vi "IMAQdx Errorcodes.vi"() -> ()   [LabVIEW 2014]
uses:
  <vilib>/Utility/error.llb/DialogType.ctl
panel:
  out "Array":errorcluster[](array[cluster])
  # "IMAQdxErrorSystemMemoryFull = 0xBFF69000,   // Not enough memory\n    IMAQdxErrorInternal,                        // Internal error\n    IMAQdxErrorInvalidParameter,                // Invalid parameter\n    IMAQdxErrorInvalidPointer,                  // Invalid pointer\n    IMAQdxErrorInvalidInterface,                // Invalid camera session\n    IMAQdxErrorInvalidRegistryKey,              // Invalid registry key\n    IMAQdxErrorInvalidAddress,                  // Invalid address\n    IMAQdxErrorInvalidDeviceType,               // Invalid device type\n    IMAQdxErrorNotImplemented,                  // Not implemented\n    IMAQdxErrorCameraNotFound,                  // Camera not found\n    IMAQdxErrorCameraInUse,                     // Camera is already in use.\n    IMAQdxErrorCameraNotInitialized,            // Camera is not initialized.\n    IMAQdxErrorCameraRemoved,                   // Camera has been removed.\n    IMAQdxErrorCameraRunning,                   // Acquisition in progress.\n    IMAQdxErrorCameraNotRunning,                // No acquisition in progress.\n    IMAQdxErrorAttributeNotSupported,           // Attribute not supported by the camera.\n    IMAQdxErrorAttributeNotSettable,            // Unable to set attribute.\n    IMAQdxErrorAttributeNotReadable,            // Unable to get attribute.\n    IMAQdxErrorAttributeOutOfRange,             // Attribute value is out of range.\n    IMAQdxErrorBufferNotAvailable,              // Requested buffer is unavailable.\n    IMAQdxErrorBufferListEmpty,                 // Buffer list is empty. Add one or more buffers.\n    IMAQdxErrorBufferListLocked,                // Buffer list is already locked. Reconfigure acquisition and try again.\n    IMAQdxErrorBufferListNotLocked,             // No buffer list. Reconfigure acquisition and try again.\n    IMAQdxErrorResourcesAllocated,              // Transfer engine resources already allocated. Reconfigure acquisition and try again.\n    IMAQdxErrorResourcesUnavailable,            // Insufficient transfer engine resources.\n    IMAQdxErrorAsyncWrite,                      // Unable to perform asychronous register write.\n    IMAQdxErrorAsyncRead,                       // Unable to perform asychronous register read.\n    IMAQdxErrorTimeout,                         // Timeout.\n    IMAQdxErrorBusReset,                        // Bus reset occurred during a transaction.\n    IMAQdxErrorInvalidXML,                      // Unable to load camera's XML file.\n    IMAQdxErrorFileAccess,                      // Unable to read/write to file.\n    IMAQdxErrorInvalidCameraURLString,          // Camera has malformed URL string.\n    IMAQdxErrorInvalidCameraFile,               // Invalid camera file.\n    IMAQdxErrorGenICamError,                    // Unknown Genicam error.\n    IMAQdxErrorFormat7Parameters,               // For format 7: The combination of speed, image position, image size, and color coding is incorrect.\n    IMAQdxErrorInvalidAttributeType,            // The attribute type is not compatible with the passed variable type.\n    IMAQdxErrorDLLNotFound,                     // The DLL could not be found.\n    IMAQdxErrorFunctionNotFound,                // The function could not be found.\n    IMAQdxErrorLicenseNotActivated,             // License not activated.\n    IMAQdxErrorCameraNotConfiguredForListener,  // The camera is not configured properly to support a listener.\n    IMAQdxErrorCameraMulticastNotAvailable,     // Unable to configure the system for multicast support.\n    IMAQdxErrorBufferHasLostPackets,            // The requested buffer has lost packets and the user requested an error to be generated.\n    IMAQdxErrorGiGEVisionError,                 // Unknown GiGE Vision error.\n    IMAQdxErrorNetworkError,                    // Unknown network error.\n    IMAQdxErrorCameraUnreachable,               // Unable to connect to the camera.\n    IMAQdxErrorHighPerformanceNotSupported,     // High performance acquisition is not supported on the specified network interface. Connect the camera to a network interface running the high performance driver.\n    IMAQdxErrorInterfaceNotRenamed,             // Unable to rename interface. Invalid or duplicate name specified.\n    IMAQdxErrorNoSupportedVideoModes,           // The camera does not have any video modes which are supported.\n    IMAQdxErrorSoftwareTriggerOverrun,          // Software trigger overrun.\n    IMAQdxErrorTestPacketNotReceived,           // The system did not receive a test packet from the camera. The packet size may be too large for the network configuration or a firewall may be enabled.\n    IMAQdxErrorCorruptedImageReceived,          // The camera returned a corrupted image.\n    IMAQdxErrorCameraConfigurationHasChanged,   // The camera did not return an image of the correct type it was configured for previously.\n    IMAQdxErrorCameraInvalidAuthentication,     // The camera is configured with password authentication and either the user name and password were not configured or they are incorrect.\n    IMAQdxErrorUnknownHTTPError,                // The camera returned an unknown HTTP error.\n    IMAQdxErrorKernelDriverUnavailable,         // Unable to attach to the kernel mode driver.\n    IMAQdxErrorPixelFormatDecoderUnavailable,   // No decoder available for selected pixel format.\n    IMAQdxErrorFirmwareUpdateNeeded,            // The acquisition hardware needs a firmware update before it can be used.\n    IMAQdxErrorFirmwareUpdateRebootNeeded,      // The firmware on the acquisition hardware has been updated and the system must be rebooted before use.\n    IMAQdxErrorLightingCurrentOutOfRange,       // The requested current level from the lighting controller is not possible.\n    IMAQdxErrorUSB3VisionError,                 // Unknown USB3 Vision error.\n    IMAQdxErrorInvalidU3VUSBDescriptor,         // The camera has a USB descriptor that is incompatible with the USB3 Vision specification.\n    IMAQdxErrorU3VInvalidControlInterface,      // The USB3 Vision control interface is not implemented or is invalid on this camera.\n    IMAQdxErrorU3VControlInterfaceError,        // There was an error from the control interface of the USB3 Vision camera.\n    IMAQdxErrorU3VInvalidEventInterface,        // The USB3 Vision event interface is not implemented or is invalid on this camera.\n    IMAQdxErrorU3VEventInterfaceError,          // There was an error from the event interface of the USB3 Vision camera.\n    IMAQdxErrorU3VInvalidStreamInterface,       // The USB3 Vision stream interface is not implemented or is invalid on this camera.\n    IMAQdxErrorU3VStreamInterfaceError,         // There was an error from the stream interface of the USB3 Vision camera.\n    IMAQdxErrorU3VUnsupportedConnectionSpeed,   // The USB connection speed is not supported by the camera.  Check whether the camera is plugged into a USB 2.0 port instead of a USB 3.0 port.  If so, verify that the camera supports this use case.       \n    IMAQdxErrorU3VInsufficientPower,            // The USB3 Vision camera requires more current than can be supplied by the USB port in use.\n    IMAQdxErrorU3VInvalidMaxCurrent,            // The U3V_MaximumCurrentUSB20_mA registry value is not valid for the connected USB3 Vision camera.\n    IMAQdxErrorBufferIncompleteData,            // The requested buffer has incomplete data and the user requested an error to be generated.\n    IMAQdxErrorCameraAcquisitionConfigFailed,   // The camera returned an error starting the acquisition.\n    IMAQdxErrorCameraClosePending,              // The camera still has outstanding references and will be closed when these operations complete.\n    IMAQdxErrorSoftwareFault,                   // An unexpected software error occurred.\n    IMAQdxErrorCameraPropertyInvalid,           // The value for an invalid camera property was requested.\n    IMAQdxErrorJumboFramesNotEnabled,           // Jumbo frames are not enabled on the host.  Maximum packet size is 1500 bytes.\n    IMAQdxErrorBayerPixelFormatNotSelected,     // This operation requires that the camera has a Bayer pixel format selected."
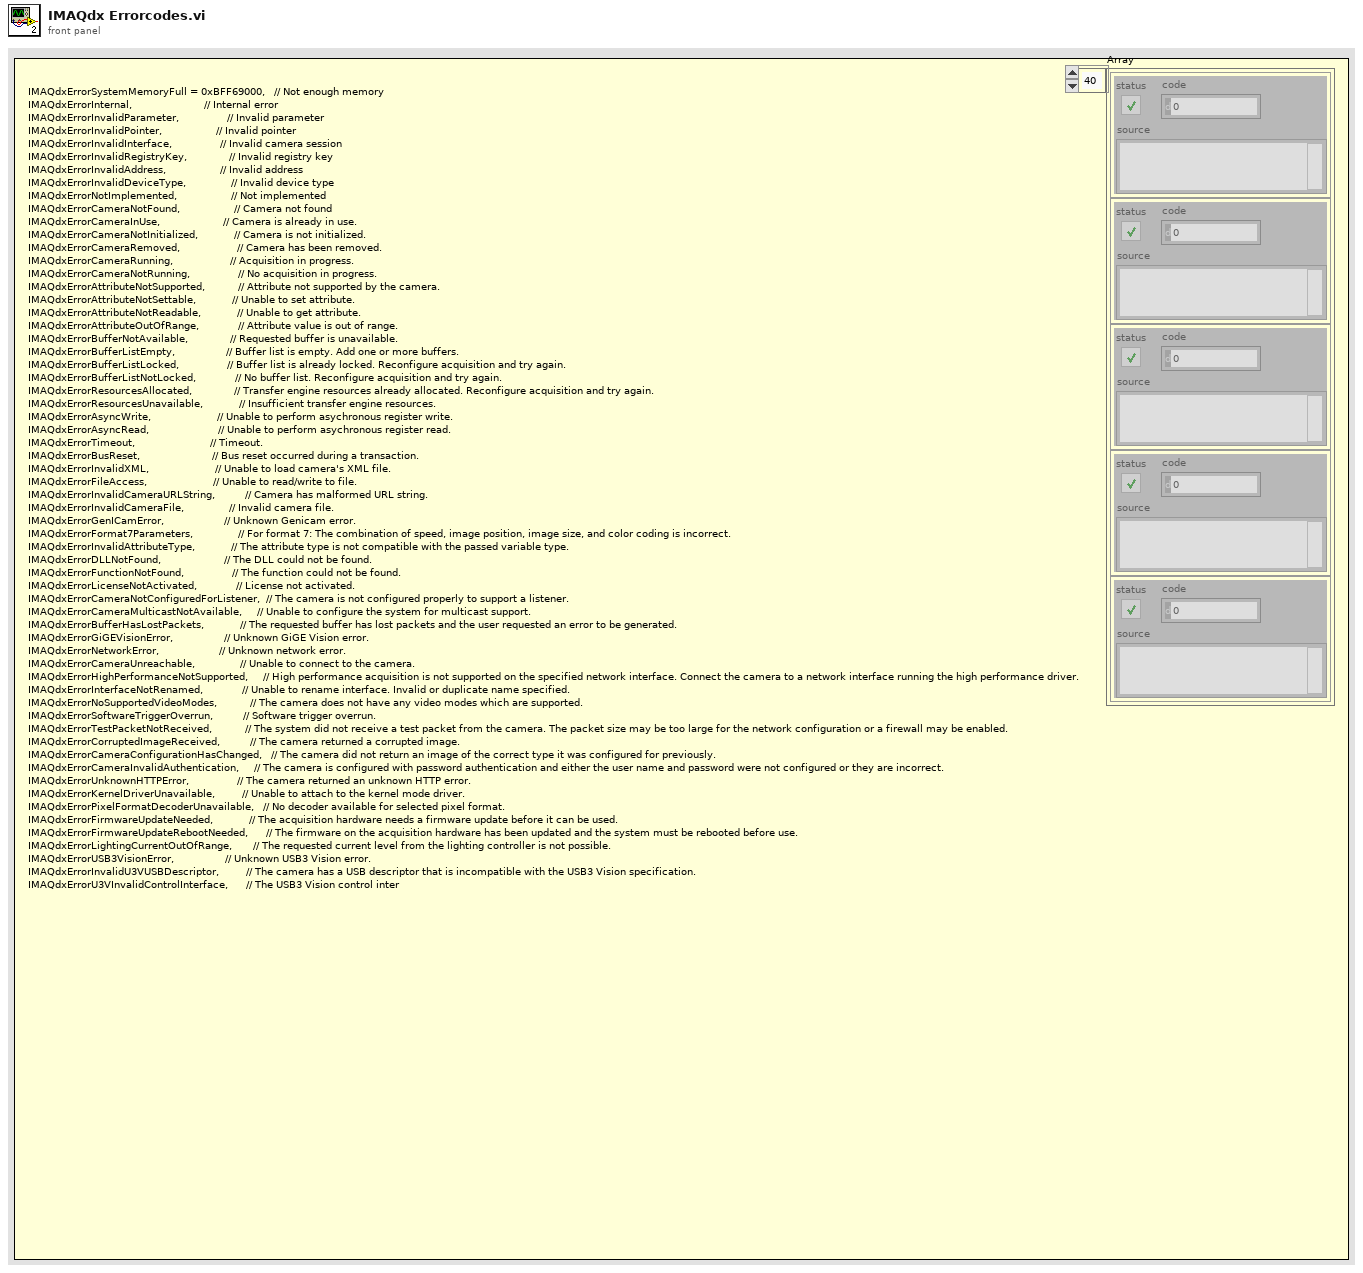
[diagram p1: front panel]
types:
  T1 = typedef "DialogType.ctl" = u16
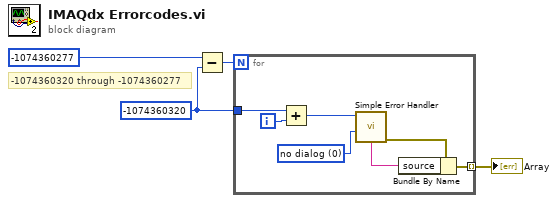
[diagram p0: block diagram]
diagram:
  w2 = -1074360320
  # "-1074360320 through -1074360277"
  n1 = Subtract(x=-1074360277, y=w2) -> (x-y=w3:i32)
  n2 = for {
    N: w3 -> [_]
    tunnel: w2 -> [w10]
    tunnel: [w6] -> w1 mode=indexing
    i -> [w11]
    w8 = T1 0 items=["no dialog", "OK message", "continue or stop message", "OK message + warnings", "continue/stop + warnings"] ("type of dialog (OK msg:1)")
    n3 = Add(x=w10, y=w11) -> (x+y=w9:i32)
    n4 = call <vilib>:"Simple Error Handler.vi"("error code (no error:0)"=w9, "type of dialog (OK msg:1)"=w8) -> ("error out"=w7:errorcluster, "message"=w5:string)  [unwired: 3 in, 3 out]
    n5 = Bundle By Name(cluster=w7, "source"=w5) -> (w6:errorcluster)
  }
  "Array" <- w1
